vi "Read Rank.vi"(8 "error in (no error)":errorcluster, 11 "Vector Abstract Path Group in":refnum<class "Vector Abstract Path Group.lvclass">) -> (0 "error out":errorcluster, 2 "Rank":dbl, 3 "Vector Abstract Path Group out":refnum<class "Vector Abstract Path Group.lvclass">)   [LabVIEW 2023, in "RFFixtureCharact.Public.lvlib" / "Vector Abstract Path Group.lvclass"]
uses:
  Vector Abstract Path Group.lvclass
  Vector Abstract Path Group.lvclass/Vector Abstract Path Group.ctl
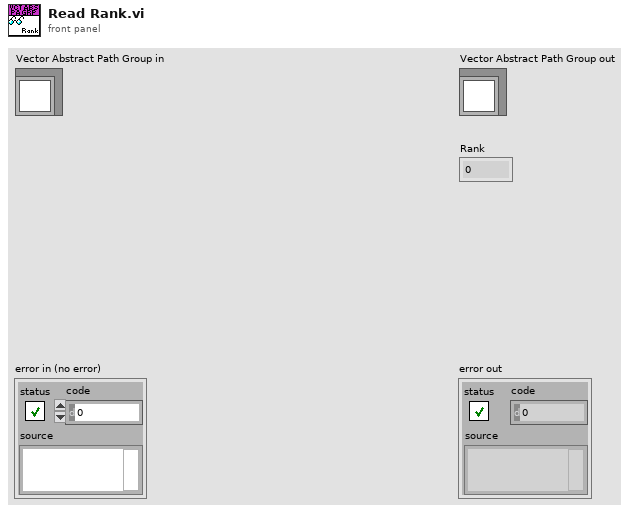
[diagram p1: front panel]
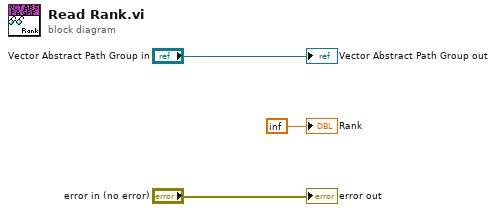
[diagram p0: block diagram]
diagram:
  "error out" <- "error in (no error)"
  "Vector Abstract Path Group out" <- "Vector Abstract Path Group in"
  "Rank" <- inf
